vi "Vision Processing.vi"(4 "error in (no error)":errorcluster, 7 "Image Size":T4=enum."320x240") -> ()   [LabVIEW 2013]
doc: "This VI runs in parallel to other tasks. It gets images from the camera, processes them for color or shape and use that information to affect robot behavior."
uses:
  <vilib>/Rock Robotics/WPI/Camera/WPI_CameraImageSize.ctl
  Robot Global Data.vi
  <vilib>/Rock Robotics/WPI/Camera/WPI_CameraFrameRate.ctl
  <vilib>/Rock Robotics/WPI/Camera/WPI_CameraExposure Values.ctl
  <vilib>/Rock Robotics/WPI/Camera/WPI_CameraWhite Balance Values.ctl
  <vilib>/vision/NI_Vision_Development_Module.lvlib
panel:
  in  "error in (no error) 2":errorcluster
  in  "Camera Name":string="Camera"
  in  "Processing":enum32{"Color", "Monochrome"}(tab)=enum."Monochrome"
  out "Value":cluster{i32, i32}
  out "Saturation":cluster{i32, i32}
  out "Hue":cluster{i32, i32}
  in  "Luminance":i32=255
  in  "Saturation 2":i32=255
  in  "Hue 2":i32(knob)=65 scale=0.0..255.0
  in  "Margins":cluster{"Hue":i32, "Sat":i32, "Val":i32}={"Hue"=33, "Sat"=53, "Val"=9} {"Sat" scale=0.0..80.0; "Val" scale=0.0..80.0; "Hue" scale=0.0..80.0}
  in  "Range":cluster{"Lower value":sgl, "Upper value":sgl}={"Lower value"=253.15218, "Upper value"=255.0} {"Upper value" scale=0.0..255.0}
  in  "Particle Count Limit":i32=8
  in  "Area Size Limit %":dbl=0.5
  in  "Score Limits":T1={"Rect Coverage"=60.0, "X Edge Strength"=40.0, "Y Edge Strength"=60.0, "Center"=75.0, "Outer"=75.0}
  in  "Camera Type":enum16{"206", "1011"}(ring)=enum."1011"
  out "Target Info":T2(array[cluster])
  out "Processed Image":T3(plugin-control)
  # "Lower/Upper"
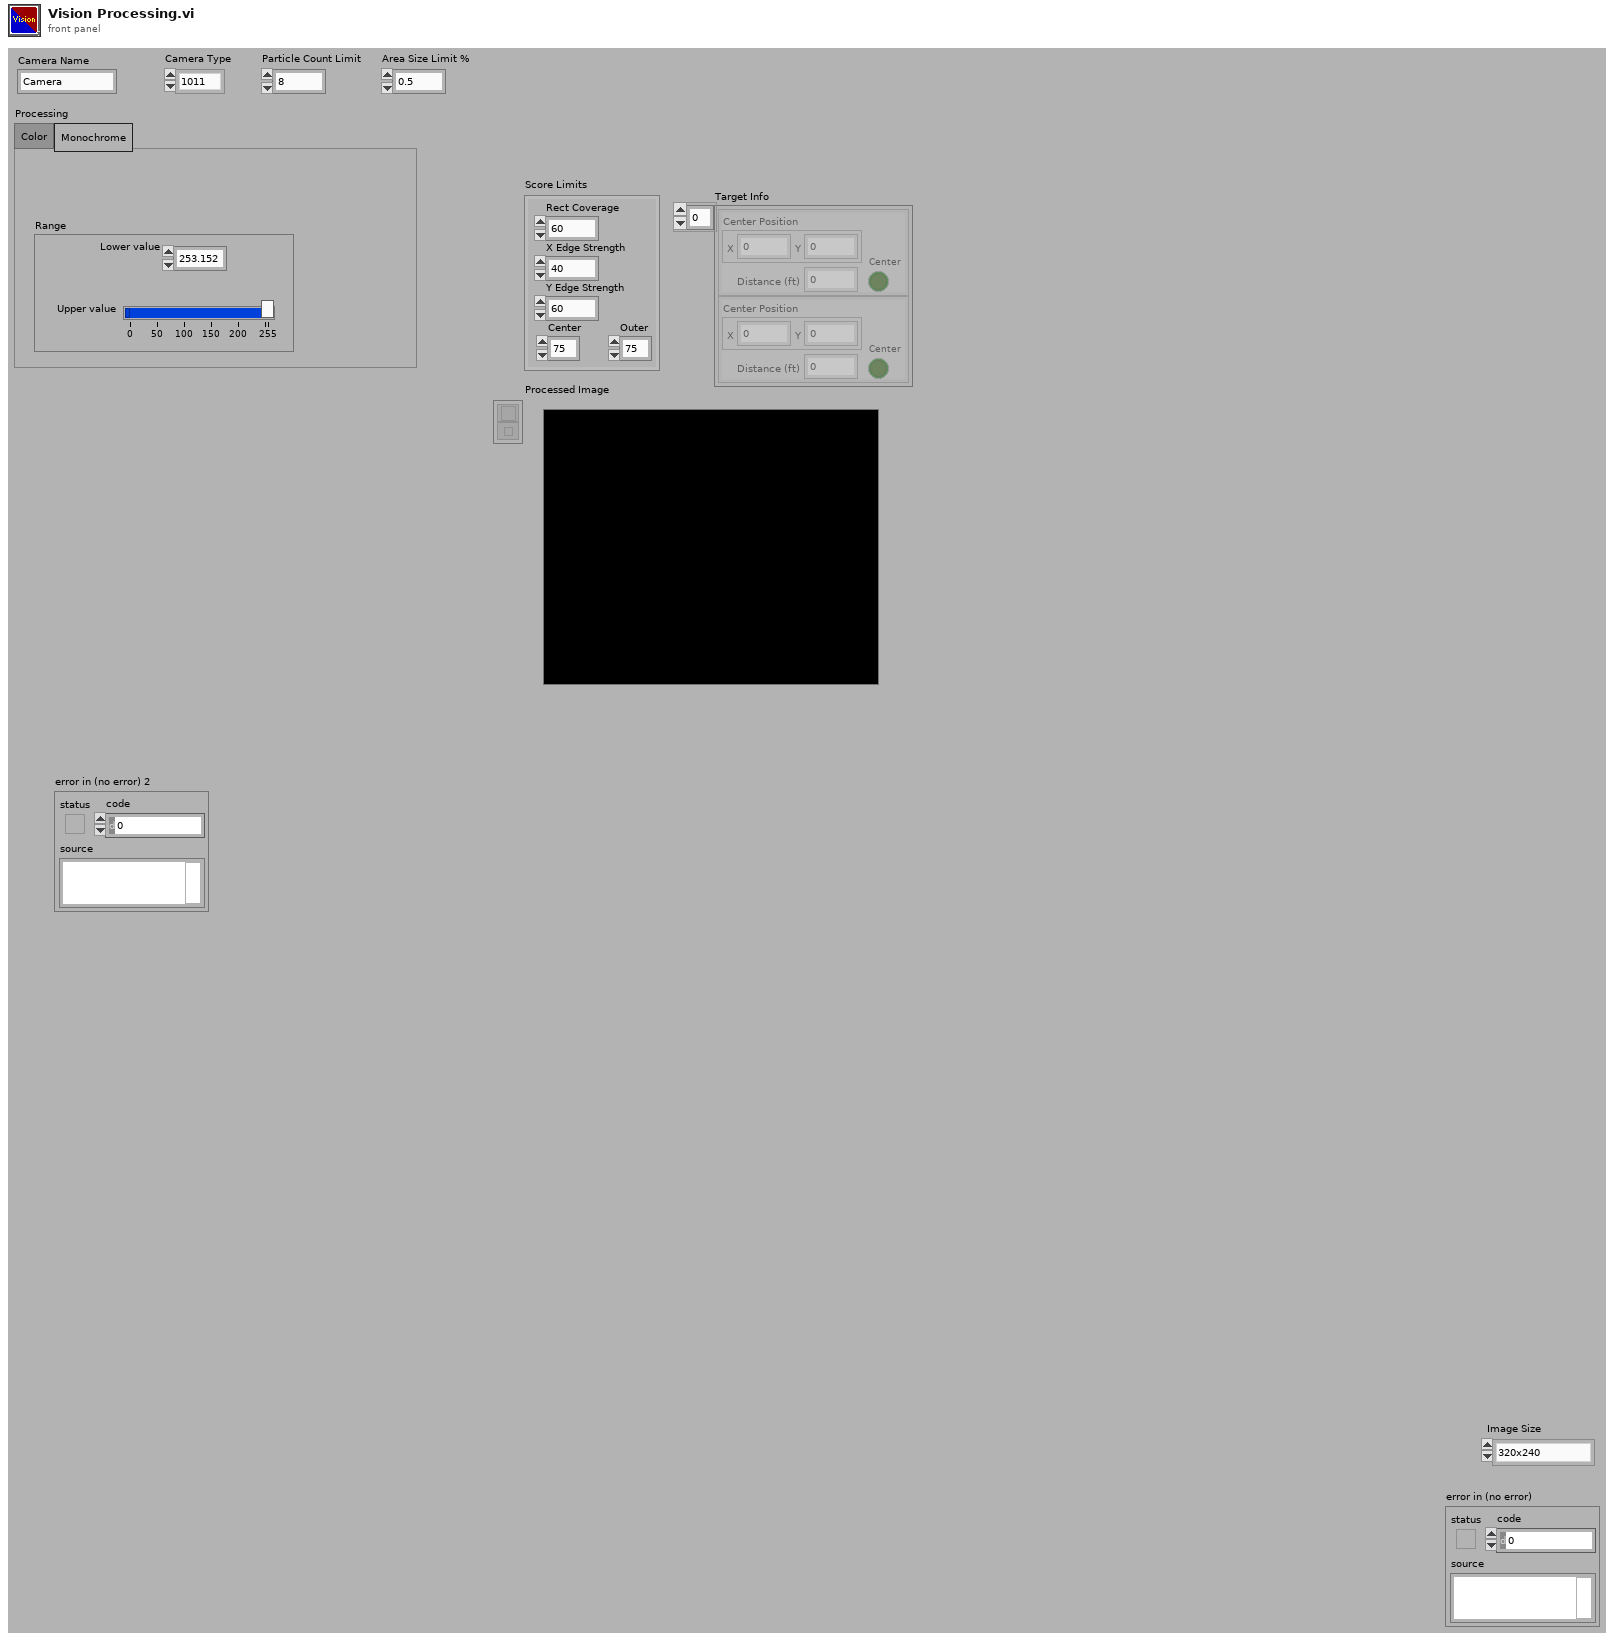
[diagram p1: front panel]
types:
  T1 = cluster{"Rect Coverage":dbl, "X Edge Strength":dbl, "Y Edge Strength":dbl, "Center":dbl, "Outer":dbl}
  T2 = cluster{"Center Position":cluster{"X":dbl, "Y":dbl}, "Distance (ft)":dbl, "Center":bool}[]
  T3 = typedef "IMAQ Image.ctl" = refnum<image>
  T4 = typedef "WPI_CameraImageSize.ctl" = enum16{"640x480", "320x240", "160x120"}
  T5 = typedef "Image Type" = u32
  T6 = typedef "WPI_CameraDevRef.ctl" = cluster{"Camera Address":string, "CameraStatus":errorcluster, "Acquire Image Notifier":refnum<notifier>}
  T7 = typedef "WPI_CameraFrameRate.ctl" = u32
  T8 = typedef "WPI_CameraExposure Values.ctl" = enum16{"Auto", "Flicker-free 50 Hz", "Flicker-free 60 Hz", "Hold current"}
  T9 = typedef "WPI_CameraWhite Balance Values.ctl" = enum16{"Auto", "Fixed indoor", "Fixed outdoor 1", "Fixed outdoor 2", "Fixed fluorescent 1", "Fixed fluorescent 2", "Hold current"}
  T10 = cluster{"Position":cluster{"X":dbl, "Y":dbl}, "Distance (ft)":dbl, "Center":bool}[]
  T11 = cluster{"Horizontal":bool, "Aspect Score":dbl, "Rect Score":dbl, cluster{"Left":dbl, "Top":dbl, "Right":dbl, "Bottom":dbl}, "Equiv H":dbl, "Equiv V":dbl}[]
  T12 = typedef "TargetType.ctl" = enum16{"Not Hot", "Hot"}
  T13 = cluster{"Scores":cluster{"Total":dbl, "Left":dbl, "Right":dbl, "Ratio":dbl, "Vertical":dbl, "index":i32, "State":T12}, "Verticals":cluster{"Horizontal?":bool, "Aspect Score":dbl, "Rect Score":dbl, cluster{"Left":dbl, "Top":dbl, "Right":dbl, "Bottom":dbl}, "Equiv H":dbl, "Equiv V":dbl}, "Horizontals":cluster{"Horizontal?":bool, "Aspect Score":dbl, "Rect Score":dbl, cluster{"Left":dbl, "Top":dbl, "Right":dbl, "Bottom":dbl}, "Equiv H":dbl, "Equiv V":dbl}, "Validated":bool}[]
  T14 = cluster{"Target Center (-1 to 1)":cluster{"X":dbl, "Y":dbl}, "Distance (ft)":dbl, "Center Target":bool}
  T15 = cluster{"Target Center (-1 to 1)":cluster{"X":dbl, "Y":dbl}, "Distance (ft)":dbl, "Center Target":bool}[]
  T16 = cluster{"Position":cluster{"X":dbl, "Y":dbl}, "Distance (ft)":dbl, "Center":bool}
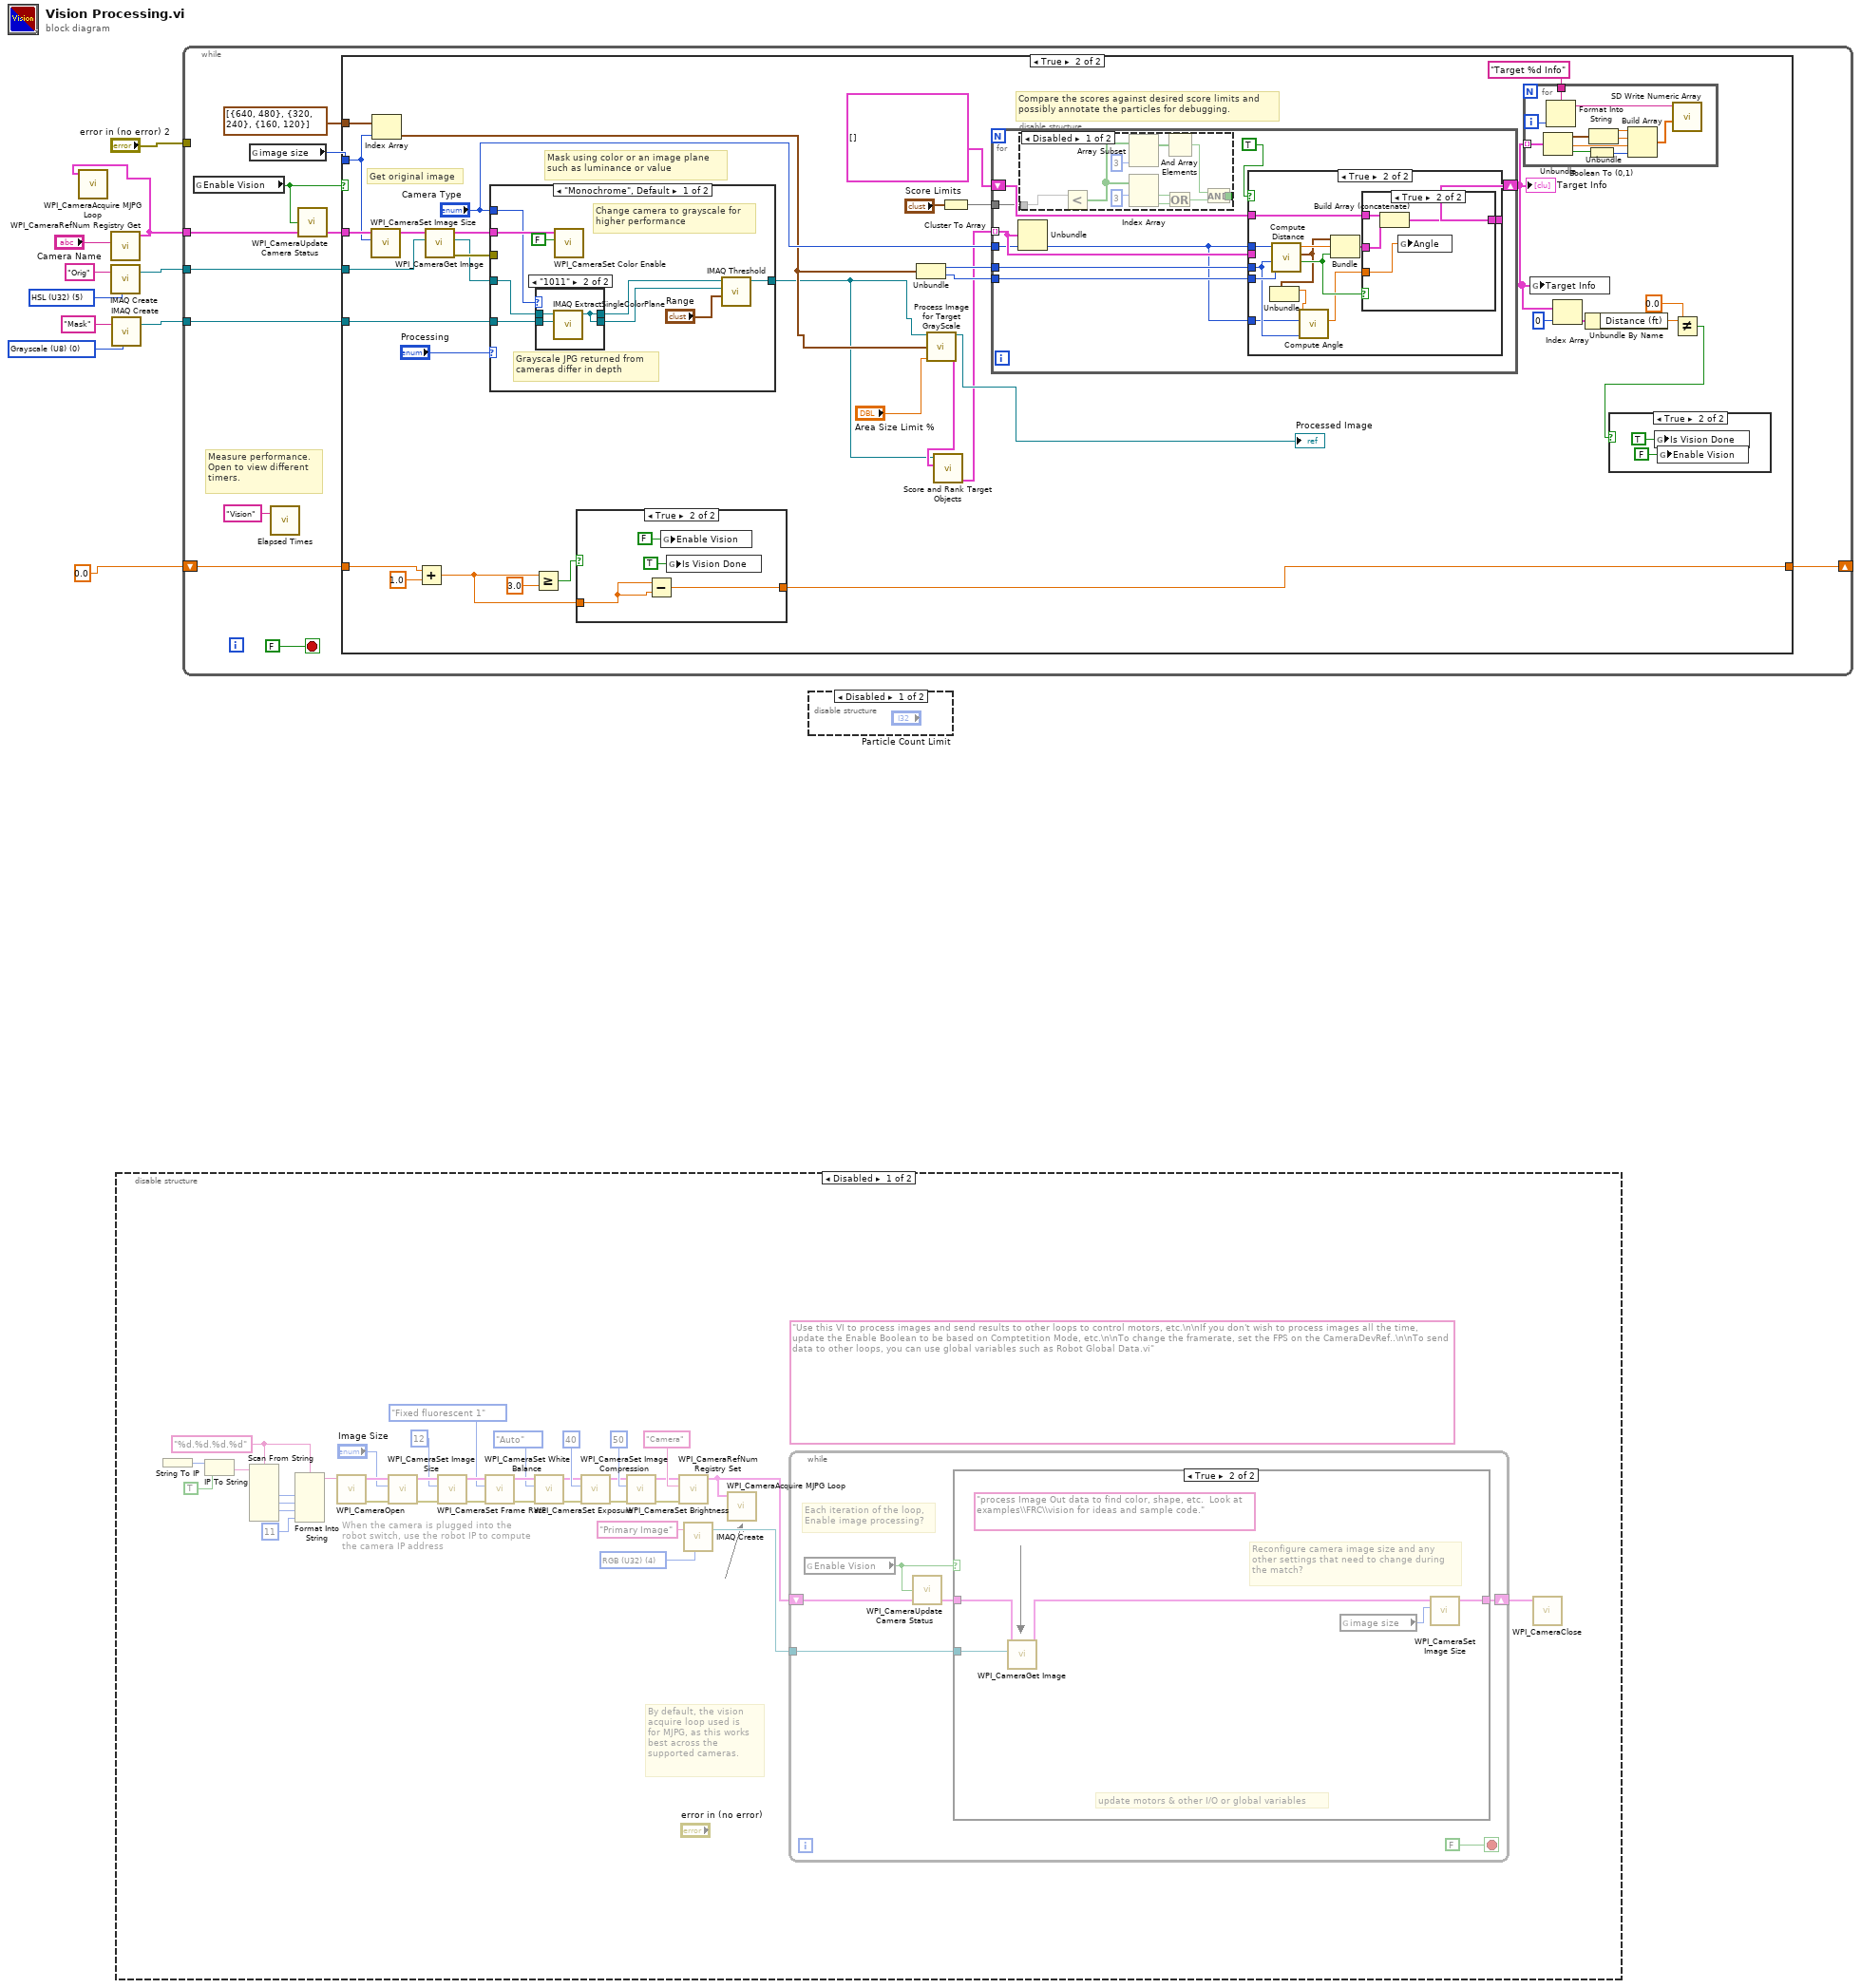
[diagram p0: block diagram]
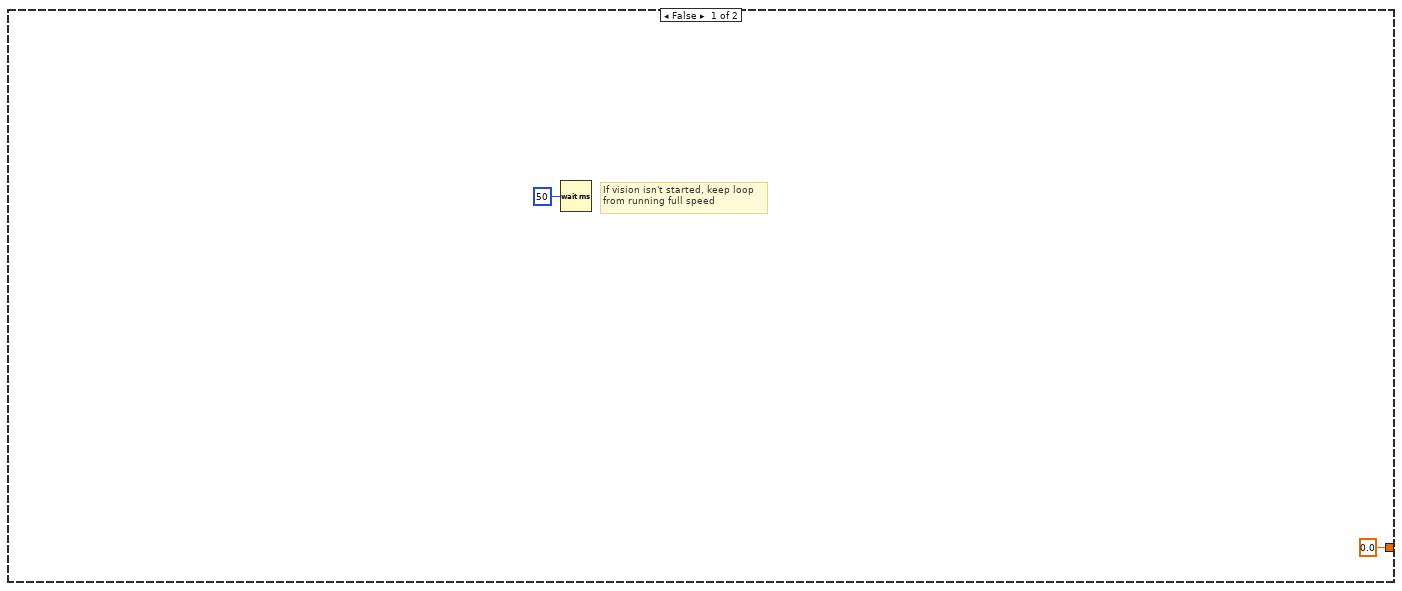
[diagram p3: hidden frame]
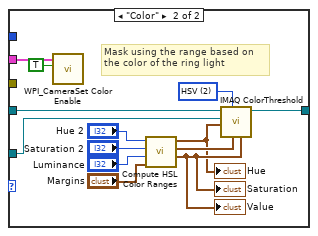
[diagram p7: hidden frame]
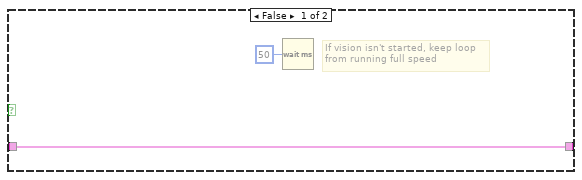
[diagram p11: hidden frame]
diagram:
  w5 = T5 0 items=["Grayscale (U8)", "Grayscale (I16)", "Grayscale (SGL)", "Complex (CSG)", "RGB (U32)", "HSL (U32)", "RGB (U64)", "Grayscale (U16)"] ("Image Type")
  w9 = T5 5 items=["Grayscale (U8)", "Grayscale (I16)", "Grayscale (SGL)", "Complex (CSG)", "RGB (U32)", "HSL (U32)", "RGB (U64)", "Grayscale (U16)"] ("Image Type")
  n1 = call <vilib>:"WPI_CameraRefNum Registry Get.vi"("refnum name"="Camera Name") -> ("CameraDevRef"=w1:T6)  [unwired: 9 in, 1 out]
  n2 = call <vilib>:"WPI_CameraAcquire MJPG Loop.vi"("CameraDevRef"=w1) -> ()  [unwired: 11 in]
  n3 = call "IMAQ Create"("Image Name"="Orig", "Image Type"=w9) -> ("New Image"=w8:T3)  [unwired: 2 in, 2 out]
  n4 = call "IMAQ Create"("Image Name"="Mask", "Image Type"=w5) -> ("New Image"=w3:T3)  [unwired: 2 in, 2 out]
  n5 = disable-structure shown="Disabled" {
    frame Disabled {
      w13 = "%d.%d.%d.%d" ("format string")
      w42 = T5 4 items=["Grayscale (U8)", "Grayscale (I16)", "Grayscale (SGL)", "Complex (CSG)", "RGB (U32)", "HSL (U32)", "RGB (U64)"] ("Image Type")
      (unwired) "Use this VI to process images and send results to other loops to control motors, etc.\n\nIf you don't wish to process images all the time, update the Enable Boolean to be based on Comptetition Mode, etc.\n\nTo change the framerate, set the FPS on the CameraDevRef..\n\nTo send data to other loops, you can use global variables such as Robot Global Data.vi"
      # "When the camera is plugged into the\nrobot switch, use the robot IP to compute\nthe camera IP address"
      # "By default, the vision\nacquire loop used is\nfor MJPG, as this works\nbest across the\nsupported cameras."
      n6 = String To IP() -> (0:w20:u32)  [unwired: 1 in]
      n7 = IP To String(1:TRUE ("dot notation? (F)"), 2:w20) -> (0:w18:string)
      n8 = Scan From String(format string=w13, input string=w18) -> (output 1=w17:i32, output 2=w16:i32, output 3=w15:i32)  [unwired: 7 in, 3 out]
      n9 = Format Into String(format string=w13, w17, w16, w15, 11 ("Compression")) -> (resulting string=w12:string)  [unwired: 2 in, 1 out]
      n10 = call <vilib>:"WPI_CameraOpen.vi"("Camera Address"=w12) -> ("error out"=w31:errorcluster, "CameraDevRef"=w32:T6)  [unwired: 1 in, 8 out]
      n11 = call <vilib>:"WPI_CameraSet Image Size.vi"("error in (no error)"=w31, "Image Size"="Image Size", "CameraDevRef"=w32) -> ("error out"=w30:errorcluster, "CameraDevRef Out"=w33:T6)  [unwired: 7 out]
      n12 = call <vilib>:"WPI_CameraSet Frame Rate.vi"("error in (no error)"=w30, "Frame Rate (fps)"=T7 12, "CameraDevRef"=w33) -> ("error out"=w29:errorcluster, "CameraDevRef Out"=w35:T6)  [unwired: 7 out]
      n13 = call <vilib>:"WPI_CameraSet White Balance.vi"("error in (no error)"=w29, "White Balance"=WPI_CameraWhite_Balance_Values."Fixed fluorescent 1", "CameraDevRef"=w35) -> ("error out"=w28:errorcluster, "CameraDevRef Out"=w34:T6)  [unwired: 7 out]
      n14 = call <vilib>:"WPI_CameraSet Exposure.vi"("error in (no error)"=w28, "Exposure"=WPI_CameraExposure_Values."Auto", "CameraDevRef"=w34) -> ("error out"=w27:errorcluster, "CameraDevRef Out"=w37:T6)  [unwired: 7 out]
      n15 = call <vilib>:"WPI_CameraSet Image Compression.vi"("error in (no error)"=w27, "Compression"=40, "CameraDevRef"=w37) -> ("error out"=w26:errorcluster, "CameraDevRef Out"=w36:T6)  [unwired: 7 out]
      n16 = call <vilib>:"WPI_CameraSet Brightness.vi"("error in (no error)"=w26, "Brightness"=50, "CameraDevRef"=w36) -> ("error out"=w24:errorcluster, "CameraDevRef Out"=w25:T6)  [unwired: 7 out]
      n17 = call <vilib>:"WPI_CameraRefNum Registry Set.vi"("error in (no error)"=w24, "refnum name"="Camera", "CameraDevRef"=w25) -> ("CameraDevRef"=w44:T6)  [unwired: 8 out]
      n18 = call "IMAQ Create"("Image Name"="Primary Image", "Image Type"=w42) -> ("New Image"=w45:T3)  [unwired: 2 in, 2 out]
      n19 = call <vilib>:"WPI_CameraAcquire MJPG Loop.vi"("CameraDevRef"=w44) -> ()  [unwired: 11 in]
      n20 = while {
        shift-right: [w50] -> w43
        shift-left: w44 -> [w48]
        tunnel: w45 -> [w49]
        stop <- FALSE stop-if-true
        # "Each iteration of the loop,\nEnable image processing?"
        n21 = global read "Robot Global Data.vi" "Enable Vision"() -> (w46:bool)
        n22 = call <vilib>:"WPI_CameraUpdate Camera Status.vi"("CameraDevRef In"=w48, "Enable Vision"=w46) -> ("CameraDevRef Out"=w47:T6)  [unwired: 3 in]
        n23 = case shown="True" w46 {
          tunnel: w49 -> [_ w57]
          tunnel: [w53 w58] -> w50
          tunnel: w47 -> [w53 w55]
          frame False {
            # "If vision isn't started, keep loop\nfrom running full speed"
            n24 = Wait (ms)(milliseconds to wait=u32 50) -> ()  [unwired: 1 out]
          }
          frame True {
            (unwired) "process Image Out data to find color, shape, etc.  Look at examples\\FRC\\vision for ideas and sample code."
            # "update motors & other I/O or global variables"
            # "Reconfigure camera image size and any\nother settings that need to change during\nthe match?"
            n25 = call <vilib>:"WPI_CameraGet Image.vi"("Image"=w57, "CameraDevRef"=w55) -> ("CameraDevRef Out"=w54:T6)  [unwired: 1 in, 8 out]
            n26 = global read "Robot Global Data.vi" "image size"() -> (w56:T4)
            n27 = call <vilib>:"WPI_CameraSet Image Size.vi"("Image Size"=w56, "CameraDevRef"=w54) -> ("CameraDevRef Out"=w58:T6)  [unwired: 1 in, 8 out]
          }
        }
      }
      n28 = call <vilib>:"WPI_CameraClose.vi"("CameraDevRef"=w43) -> ()  [unwired: 1 in, 10 out]
    }
    frame Enabled {
    }
  }
  n29 = while {
    tunnel: w8 -> [w68]
    tunnel: w1 -> [w67]
    tunnel: "error in (no error) 2" -> [_]
    tunnel: w3 -> [w62]
    shift-right: [w59] -> _
    shift-left: 0.0 -> [w60]
    stop <- FALSE stop-if-true
    # "Measure performance.\nOpen to view different\ntimers."
    n30 = global read "Robot Global Data.vi" "Enable Vision"() -> (w65:bool)
    n31 = global read "Robot Global Data.vi" "image size"() -> (w63:T4)
    n32 = call "Elapsed Times.vi"("Call Name"="Vision") -> ()  [unwired: 2 in, 1 out]
    n33 = call <vilib>:"WPI_CameraUpdate Camera Status.vi"("CameraDevRef In"=w67, "Enable Vision"=w65) -> ("CameraDevRef Out"=w66:T6)  [unwired: 3 in]
    n34 = case shown="True" w65 {
      tunnel: w68 -> [_ w103]
      tunnel: w66 -> [_ w99]
      tunnel: w63 -> [_ w98]
      tunnel: w62 -> [_ w94]
      tunnel: cluster{i32, i32}[] [{640, 480}, {320, 240}, {160, 120}] -> [_ w97]
      tunnel: w60 -> [_ w88]
      tunnel: [0.0 w84] -> w59
      frame False {
        # "If vision isn't started, keep loop\nfrom running full speed"
        n35 = Wait (ms)(milliseconds to wait=u32 50) -> ()  [unwired: 1 out]
      }
      frame True {
        # "Compare the scores against desired score limits and\npossibly annotate the particles for debugging."
        # "Mask using color or an image plane\nsuch as luminance or value"
        # "Get original image"
        n36 = call <vilib>:"WPI_CameraSet Image Size.vi"("Image Size"=w98, "CameraDevRef"=w99) -> ("CameraDevRef Out"=w100:T6)  [unwired: 8 in, 1 out]
        n37 = Index Array(array=w97, index=w98) -> (element=w77:cluster{i32, i32})
        n38 = Add(x=w88, y=1.0) -> (x+y=w85:dbl)
        n39 = call <vilib>:"WPI_CameraGet Image.vi"("Image"=w103, "CameraDevRef"=w100) -> ("error out"=w101:errorcluster, "Image Out"=w93:T3, "CameraDevRef Out"=w102:T6)  [unwired: 7 in]
        n40 = case shown="\"Monochrome\", Default" "Processing" {
          tunnel: w93 -> [w129 w151]
          tunnel: [w132 w150] -> w73
          tunnel: w102 -> [w130 w143]
          tunnel: w101 -> [_ _]
          tunnel: w94 -> [w128 w141]
          tunnel: "Camera Type" -> [w127 _]
          frame "Monochrome", Default {
            # "Grayscale JPG returned from\ncameras differ in depth"
            # "Change camera to grayscale for\nhigher performance"
            n41 = case shown="\"1011\"" w127 {
              tunnel: w129 -> [w135 w138]
              tunnel: w128 -> [w134 w137]
              tunnel: [w135 w136] -> w126
              tunnel: [w134 w136] -> w125
              frame "206", Default {
              }
              frame "1011" {
                n42 = call "IMAQ ExtractSingleColorPlane"("Image Dst"=w137, "Image Src"=w138) -> ("Image Dst Out"=w136:T3)  [unwired: 8 in, 1 out]
              }
            }
            n43 = call <vilib>:"WPI_CameraSet Color Enable.vi"("Color Enabled"=FALSE, "CameraDevRef"=w130) -> ()  [unwired: 8 in, 2 out]
            n44 = call "IMAQ Threshold"("Range"="Range", "Image Dst"=w125, "Image Src"=w126) -> ("Image Dst Out"=w132:T3)  [unwired: 3 in, 5 out]
          }
          frame "Color" {
            w149 = u16 2 items=["RGB", "HSL", "HSV", "HSI"] ("Color Mode")
            # "Mask using the range based on\nthe color of the ring light"
            n45 = call <vilib>:"WPI_CameraSet Color Enable.vi"("Color Enabled"=TRUE, "CameraDevRef"=w143) -> ()  [unwired: 8 in, 2 out]
            n46 = call "Compute HSL Color Ranges.vi"("Margins"="Margins", "Luminance"="Luminance", "Saturation"="Saturation 2", "Hue"="Hue 2") -> ("Lum Range"=w140:cluster{i32, i32}, "Sat Range"=w148:cluster{i32, i32}, "Hue Range"=w139:cluster{i32, i32})  [unwired: 5 in]
            "Hue" <- w139
            "Saturation" <- w140
            "Value" <- w140
            n47 = call "IMAQ ColorThreshold"("Blue or Luma or Val or Inten Range"=w140, "Green or Sat Range"=w148, "Color Mode"=w149, "Red or Hue Range"=w139, "Image Dst"=w141, "Image Src"=w151) -> ("Image Dst Out"=w150:T3)  [unwired: 4 in, 1 out]
          }
        }
        n48 = Greater Or Equal?(x=w85, y=3.0) -> (x >= y?=w86:bool)
        n49 = case shown="True" w86 {
          tunnel: w85 -> [w109 w112]
          tunnel: [w109 w111] -> w84
          frame False {
          }
          frame True {
            n50 = Subtract(x=w112, y=w112) -> (x-y=w111:dbl)
            n51 = global write "Robot Global Data.vi" "Enable Vision"(FALSE ("Enable Vision")) -> ()
            n52 = global write "Robot Global Data.vi" "Is Vision Done"(TRUE ("Is Vision Done")) -> ()
          }
        }
        n53 = Unbundle(w77) -> (w96:i32, w95:i32)
        n54 = call "Process Image for Target GrayScale.vi"("Src Image"=w73, "Range"=w77, "Area Cutoff %"="Area Size Limit %") -> ("Src Image Out"=→"Processed Image":T3, "Particles"=w74:T11)  [unwired: 10 in, 1 out]
        n55 = call "Score and Rank Target Objects.vi"("Particles"=w74, "Image in"=w73) -> ("Target Info"=w72:T13)  [unwired: 8 in, 1 out]
        n56 = Cluster To Array(cluster="Score Limits") -> (array=w104:dbl[])
        n57 = for {
          shift-right: [w158] -> w83
          shift-left: T10 [] -> [w159]
          tunnel: w96 -> [w157]
          tunnel: w72 -> [w154] mode=indexing
          tunnel: w104 -> [w156]
          tunnel: "Camera Type" -> [w153]
          tunnel: w95 -> [w155]
          n58 = Unbundle(w154) -> ()  [unwired: 4 out]
          n59 = disable-structure shown="Disabled" {
            disable-tunnel: w156 -> [w169 _]
            disable-tunnel: [w160 _] -> _
            frame Disabled {
              n60 = Less?(x=w169) -> (x < y?=w161:bool[])  [unwired: 1 in]
              n61 = Array Subset(array=w161, length=3) -> (w163:bool[])  [unwired: 1 in]
              n62 = Index Array(array=w161, index #1=3 ("length")) -> (element #1=w165:bool, element #2=w166:bool)  [unwired: 1 in]
              n63 = And Array Elements(Boolean array=w163) -> (logical AND=w168:bool)
              n64 = Or(x=w165, y=w166) -> (x .or. y?=w167:bool)
              n65 = And(x=w168, y=w167) -> (x .and. y?=w160:bool)
            }
            frame Enabled {
            }
          }
          n66 = case shown="True" TRUE {
            tunnel: w159 -> [w170 w182]
            tunnel: [w170 w181] -> w158
            tunnel: w157 -> [_ w175]
            tunnel: w153 -> [_ w178]
            tunnel: w155 -> [_ w177]
            tunnel: w154 -> [_ _]
            tunnel: w153 -> [_ w174]
            frame False {
            }
            frame True {
              n67 = call "Compute Distance.vi"("Y Image Resolution"=w177, "X Image Resolution"=w175, "Camera Type"=w178) -> ("Center Target"=w176:bool, "Target Center (-1 to 1)"=w173:cluster{"X":dbl, "Y":dbl}, "Distance (ft)"=w179:dbl)  [unwired: 6 in]
              n68 = Unbundle(w173) -> ("X"=w172:dbl)  [unwired: 1 out]
              n69 = call "Compute Angle.vi"("X Resolution"=w175, "Camera Type"=w174, "X Center (Relative)"=w172) -> ("Angle"=w171:dbl)  [unwired: 8 in]
              n70 = Bundle("Target Center (-1 to 1)"=w173, "Distance (ft)"=w179, "Center Target"=w176) -> (w180:T14)  [unwired: 1 in]
              n71 = case shown="True" w176 {
                tunnel: w182 -> [w183 w187]
                tunnel: [w183 w186] -> w181
                tunnel: w180 -> [_ w185]
                tunnel: w171 -> [_ w184]
                frame False {
                }
                frame True {
                  n72 = Build Array (concatenate)(w187, w185) -> (w186:T15)
                  n73 = global write "Robot Global Data.vi" "Angle"(w184) -> ()
                }
              }
            }
          }
        }
        "Target Info" <- w83
        n74 = for {
          tunnel: w83 -> [w124] mode=indexing
          tunnel: "Target %d Info" ("Name") -> [w123]
          i -> [w120]
          n75 = Unbundle(w124) -> ("Position"=w121:cluster{"X":dbl, "Y":dbl}, "Distance (ft)"=w116:dbl, "Center"=w119:bool)
          n76 = Format Into String(format string=w123, w120) -> (resulting string=w122:string)  [unwired: 2 in, 1 out]
          n77 = Boolean To (0,1)(Boolean=w119) -> (0, 1=w115:i16)
          n78 = Unbundle(w121) -> ("X"=w118:dbl, "Y"=w117:dbl)
          n79 = Build Array(w118, w117, w116, w115) -> (w114:dbl[])
          n80 = call <vilib>:"SD Write Numeric Array.vi"("Numeric Array"=w114, "Name"=w122) -> ()  [unwired: 8 in, 2 out]
        }
        n81 = global write "Robot Global Data.vi" "Target Info"(w83) -> ()
        n82 = Index Array(array=w83, index=0) -> (element=w81:T16)
        n83 = Unbundle By Name(w81) -> ("Distance (ft)"=w80:dbl)
        n84 = Not Equal?(x=w80, y=0.0) -> (x != y?=w78:bool)
        n85 = case shown="True" w78 {
          frame False {
          }
          frame True {
            n86 = global write "Robot Global Data.vi" "Is Vision Done"(TRUE ("Is Vision Done")) -> ()
            n87 = global write "Robot Global Data.vi" "Enable Vision"(FALSE ("Enable Vision")) -> ()
          }
        }
      }
    }
  }
  n88 = disable-structure shown="Disabled" {
    frame Disabled {
    }
    frame Enabled {
    }
  }
